vi "Configuration Set Von.vi"(0 "VISA resource name":refnum<visa-resource-name>, 5 "Von (1.0 V)":sgl=1.0 min=0 format="%.2f", 7 "Latch (T: On)":bool, 11 "error in (no error)":errorcluster) -> (4 "VISA resource name out":refnum<visa-resource-name>, 15 "error out":errorcluster)   [LabVIEW 2015, in "Chroma ATE 6310.lvlib"]
doc: "Set voltage of sink current on.And set the action type of Von.\n\nBe careful to select the valid voltage value,or maybe it will cause some damage."
uses:
  <instrlib>/Chroma ATE 6310/Chroma ATE 6310.lvlib
panel:
  # "On\nOff"
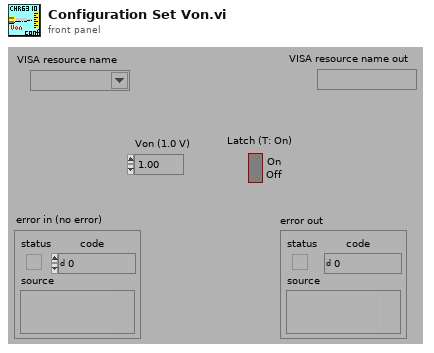
[diagram p1: front panel]
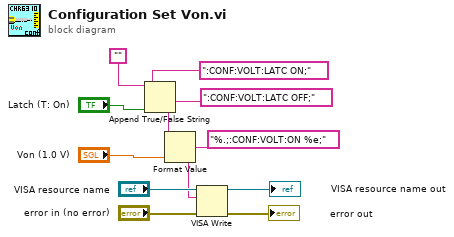
[diagram p0: block diagram]
diagram:
  n1 = Append True/False String(1:"Latch (T: On)", 2:":CONF:VOLT:LATC OFF;", 3:":CONF:VOLT:LATC ON;", 4:"") -> (0:w1:string)
  n2 = Format Value(string ("")=w1, format string="%.;:CONF:VOLT:ON %e;", value (0)="Von (1.0 V)") -> (output string=w6:string)
  n3 = VISA Write(VISA resource name="VISA resource name", write buffer=w6, error in (no error)="error in (no error)") -> (VISA resource name out=→"VISA resource name out":refnum<visa-resource-name>, error out=→"error out":errorcluster)  [unwired: 1 out]
